vi "GetOperationMeasuringRegister.vi"(8 "Error In":errorcluster, 10 "Register":T1, 11 "Kiethley 2602 In":refnum<visa-resource-name>) -> (0 "Error Out":errorcluster, 2 "Operation Measuring Register":bool[](array[boolean]), 3 "Keithley 2602 Out":refnum<visa-resource-name>)   [LabVIEW 2012, in "Keithley-2602.lvlib"]
uses:
  Keithley-2602.lvlib
  Controls/Register.ctl
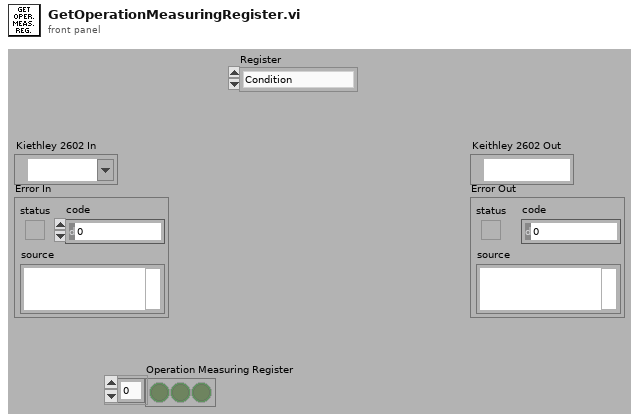
[diagram p1: front panel]
types:
  T1 = typedef "Keithley-2602.lvlib/Register.ctl" = enum16{"Condition", "Event", "Enable", "Positive Transition", "Negative Transition"}
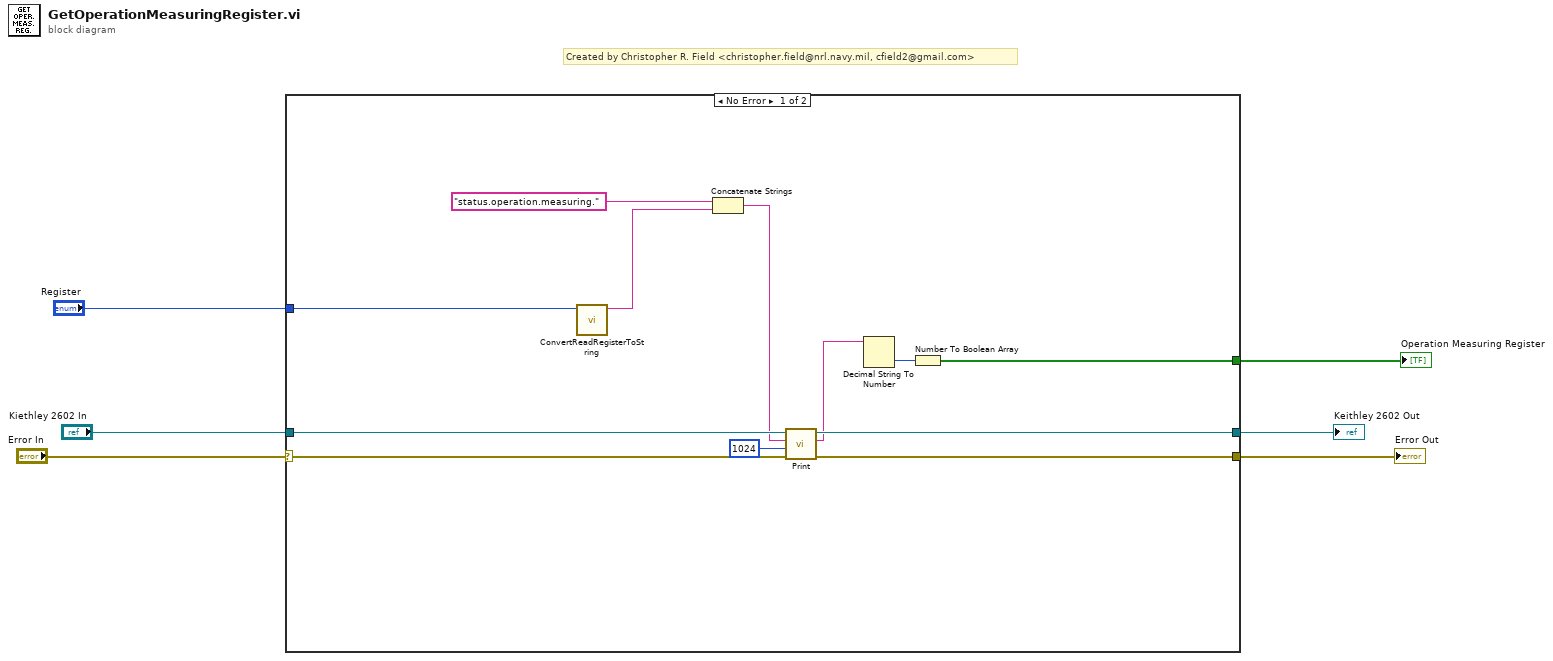
[diagram p0: block diagram]
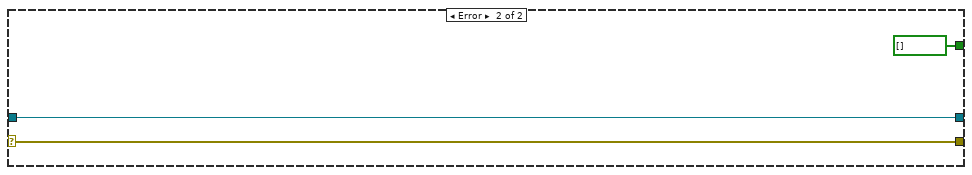
[diagram p2: hidden frame]
diagram:
  # "Created by Christopher R. Field <christopher.field@nrl.navy.mil, cfield2@gmail.com>"
  n1 = case shown="No Error" "Error In" {
    selector: "Error In" -> [w7 w21]
    tunnel: "Kiethley 2602 In" -> [w18 w20]
    tunnel: [w16 w20] -> w5
    tunnel: [w15 w21] -> w4
    tunnel: [w12 bool[] [] ("Boolean array")] -> w3
    tunnel: "Register" -> [w8 _]
    frame No Error {
      n2 = call "ConvertReadRegisterToString.vi"("Register"=w8) -> ("Register"=w9:string)  [unwired: 10 in]
      n3 = Concatenate Strings("status.operation.measuring.", w9) -> (w10:string)
      n4 = call "Print.vi"("Error In"=w7, "Byte Count"=u32 1024, "Attribute"=w10, "Kiethley 2602 In"=w18) -> ("Error Out"=w15:errorcluster, "Output"=w14:string, "Keithley 2602 Out"=w16:refnum<visa-resource-name>)  [unwired: 5 in]
      n5 = Decimal String To Number(string=w14) -> (number=w13:i32)  [unwired: 2 in, 1 out]
      n6 = Number To Boolean Array(number=w13) -> (Boolean array=w12:bool[])
    }
    frame Error {
    }
  }
  "Keithley 2602 Out" <- w5
  "Error Out" <- w4
  "Operation Measuring Register" <- w3
